vi "Set Delay Interval.vi"(8 "error in":errorcluster, 10 "Delay In":u8, 11 "Vaisala in":refnum<class "Vaisala.lvclass">) -> (0 "error out":errorcluster, 3 "Vaisala out":refnum<class "Vaisala.lvclass">)   [LabVIEW 2014, in "Vaisala Library.lvlib" / "Vaisala.lvclass"]
uses:
  Vaisala.lvclass
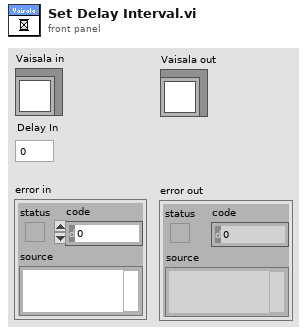
[diagram p1: front panel]
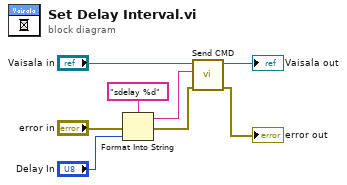
[diagram p0: block diagram]
diagram:
  n1 = Format Into String(format string="sdelay %d", error in="error in", "Delay In") -> (resulting string=w3:string, error out=w1:errorcluster)  [unwired: 1 in]
  n2 = call "Send CMD.vi"("error in"=w1, "CMD In"=w3, "Vaisala in"="Vaisala in") -> ("error out"=→"error out":errorcluster, "Vaisala out"=→"Vaisala out":refnum<class "Vaisala.lvclass">)  [unwired: 7 in]
